vi "Plot XY.vi"(8 "error in (no error)":errorcluster, 10 "Channel":u8, 11 "Instrument Actor in":refnum<class "Instrument Actor.lvclass">) -> (0 "error out":errorcluster, 3 "Instrument Actor out":refnum<class "Instrument Actor.lvclass">)   [LabVIEW 2024, in "Instrument Actor.lvclass"]
uses:
  Instrument Actor.lvclass
  Instrument Actor.lvclass/Instrument Actor.ctl
  NHMFL_Core/Libraries/Instruments/Instrument Driver/Instrument Driver.lvclass
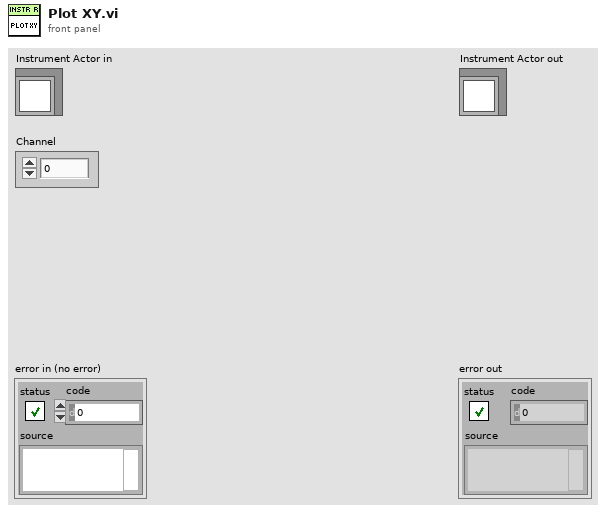
[diagram p1: front panel]
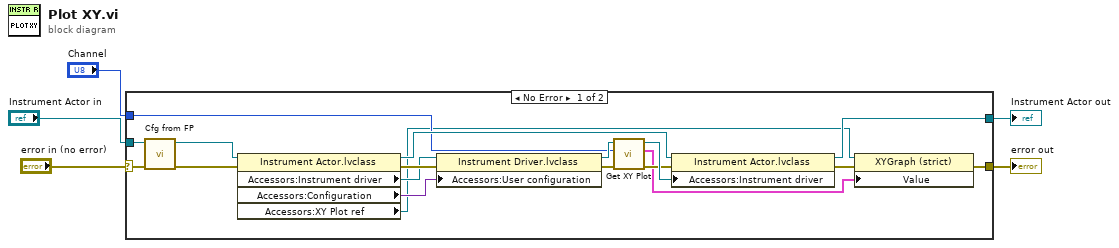
[diagram p0: block diagram]
diagram:
  n1 = case shown="No Error" "error in (no error)" {
    selector: "error in (no error)" -> [w14 w25]
    tunnel: [w17 w25] -> w2
    tunnel: [w21 w24] -> w3
    tunnel: "Instrument Actor in" -> [w15 w24]
    tunnel: "Channel" -> [w7 _]
    frame No Error {
      n2 = call-dynamic "Cfg from FP.vi"("error in (no error)"=w14, "Measure Object in"=w15) -> ("error out"=w13:errorcluster, "Measure Object out"=w12:refnum<class "Instrument Actor.lvclass">)  [unwired: 8 in]
      n3 = property class="Instrument Actor.lvclass"(reference=w12, error in=w13) -> (reference out=w18:refnum<class "Instrument Actor.lvclass">, error out=w23:errorcluster, "Accessors:Instrument driver"=w10:refnum<class "Instrument Driver.lvclass">, "Accessors:Configuration"=w8:variant, "Accessors:XY Plot ref"=w6:refnum<vi>)
      n4 = property class="Instrument Driver.lvclass"(reference=w10, error in=w23, "Accessors:User configuration"=w8) -> (reference out=w9:refnum<class "Instrument Driver.lvclass">, error out=w11:errorcluster)
      n5 = call-dynamic "Get XY Plot.vi"("error in (no error)"=w11, "Channel"=w7, "Instrument Driver in"=w9) -> ("error out"=w19:errorcluster, "XY Plot"=w16:cluster{dbl[], "Spectrum, db":dbl[]}[], "Instrument Driver out"=w20:refnum<class "Instrument Driver.lvclass">)  [unwired: 6 in]
      n6 = property class="Instrument Actor.lvclass"(reference=w18, error in=w19, "Accessors:Instrument driver"=w20) -> (reference out=w21:refnum<class "Instrument Actor.lvclass">, error out=w22:errorcluster)
      n7 = property class="XYGraph (strict)"(reference=w6, error in=w22, "Value"=w16) -> (error out=w17:errorcluster)  [unwired: 1 out]
    }
    frame Error {
    }
  }
  "error out" <- w2
  "Instrument Actor out" <- w3
